vi ".INI READ.vi"(11 "KEY":string) -> (0 "COM":string, 1 "MODE":string, 2 "TEST MODE":string, 3 "OUT":dbl, 4 "TIME":dbl, 6 "AUTH KEY":string, 8 "error out":errorcluster, 10 "Serail No":cluster{"Serial Number":T1})   [LabVIEW 2024]
uses:
  SERIAL N0.ctl
  <vilib>/Utility/config.llb/Read Key (Double).vi
  <vilib>/Utility/config.llb/Read Key (String).vi
  <vilib>/Utility/config.llb/NI_LVConfig.lvlib
panel:
  in  "Serial No 2":cluster{"Serial Number":T1}
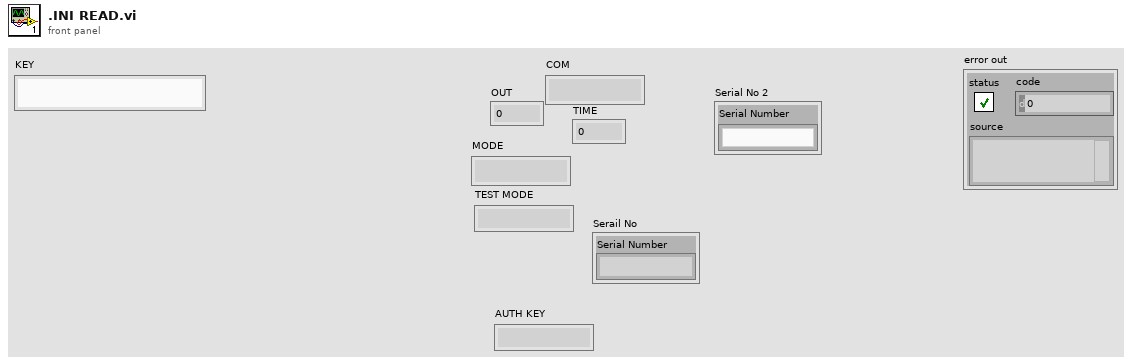
[diagram p1: front panel]
types:
  T1 = typedef "SERIAL N0.ctl" = string
  T2 = typedef "NI_LVConfig.lvlib/Config Data RefNum.ctl" = refnum<k1>
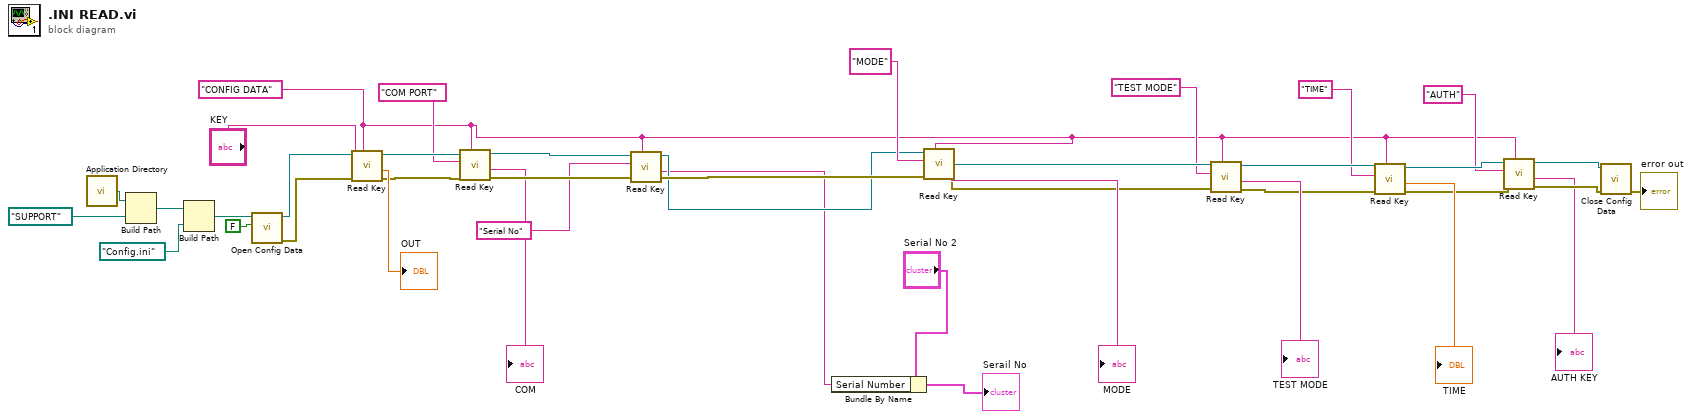
[diagram p0: block diagram]
diagram:
  w7 = "CONFIG DATA" ("section")
  n1 = call <vilib>:"Application Directory.vi"() -> ("Application Directory"=w38:path)
  n2 = Build Path(base path=w38, name or relative path=path "SUPPORT") -> (appended path=w39:path)
  n3 = Build Path(base path=w39, name or relative path=path "Config.ini") -> (appended path=w33:path)
  n4 = call <vilib>:"Open Config Data.vi"("create file if necessary (T)"=FALSE, "configuration file path"=w33) -> ("error out"=w34:errorcluster, "refnum"=w35:T2)  [unwired: 7 in, 1 out]
  n5 = call-poly <vilib>:"Read Key.vi"("section"=w7, "error in (no error)"=w34, "key"="KEY", "refnum"=w35) -> ("error out"=w28:errorcluster, "value"=→"OUT":dbl, "refnum out"=w29:T2)  [unwired: 4 in, 1 out]
  n6 = call-poly <vilib>:"Read Key.vi"("section"=w7, "error in (no error)"=w28, "key"="COM PORT", "refnum"=w29) -> ("error out"=w26:errorcluster, "value"=→"COM":string, "refnum out"=w5:T2)  [unwired: 4 in, 1 out]
  n7 = call-poly <vilib>:"Read Key.vi"("section"=w7, "key"="Serial No", "refnum"=w5) -> ("value"=w2:string, "refnum out"=w4:T2)  [unwired: 5 in, 2 out]
  n8 = Bundle By Name(cluster="Serial No 2", "Serial Number"=w2) -> (→"Serail No":cluster{"Serial Number":T1})
  n9 = call-poly <vilib>:"Read Key.vi"("section"=w7, "error in (no error)"=w26, "key"="MODE", "refnum"=w4) -> ("error out"=w21:errorcluster, "value"=→"MODE":string, "refnum out"=w22:T2)  [unwired: 4 in, 1 out]
  n10 = call-poly <vilib>:"Read Key.vi"("section"=w7, "error in (no error)"=w21, "key"="TEST MODE", "refnum"=w22) -> ("error out"=w17:errorcluster, "value"=→"TEST MODE":string, "refnum out"=w18:T2)  [unwired: 4 in, 1 out]
  n11 = call-poly <vilib>:"Read Key.vi"("section"=w7, "error in (no error)"=w17, "key"="TIME", "refnum"=w18) -> ("error out"=w13:errorcluster, "value"=→"TIME":dbl, "refnum out"=w14:T2)  [unwired: 4 in, 1 out]
  n12 = call-poly <vilib>:"Read Key.vi"("section"=w7, "error in (no error)"=w13, "key"="AUTH", "refnum"=w14) -> ("error out"=w12:errorcluster, "value"=→"AUTH KEY":string, "refnum out"=w11:T2)  [unwired: 4 in, 1 out]
  n13 = call <vilib>:"Close Config Data.vi"("error in (no error)"=w12, "refnum"=w11) -> ("error out"=→"error out":errorcluster)  [unwired: 8 in, 1 out]
